vi "Configuration File.vi"(4 "Freq List File":path, 5 "Limit File":path, 6 "Configurtion File":path, 7 "Mode (F-Read)":bool, 8 "Error In":errorcluster, 9 "Limit":T1, 10 "Freq List In":cluster{"Freq":dbl, "Amp":dbl}[](array[cluster]), 11 "Configuration":T2={"PSU Setting"={"Channel Name"="1", "Source Delay (Sec)"=0.5, "Measurement:Sense"=1008, "voltage level"=0.0, "voltage level range"=20.0, "current limit"=0.02, "current limit range"=0.02, "resource name"="PSU"}, "Sweep Settings"={"Input Settings"={"IEPE min time to settle [s]"=0.0, "Responce Channel Settings"={"DSA response channel settings"={"coupling"=10045, "enable IEPE excitation"=FALSE, "IEPE current [mA]"=4.0}, "response channel info"={"sensor sensitivity"=1000.0, "engineering units"=1, "dB reference"=1.0, "custom label"="EU", "weighting filter"=0, "pregain"=0.0}, "AI response settings"={"response channel"="SOUNDACQ/ai1", "max value [V]"=10.0, "min value [V]"=-10.0, "terminal configuration"=-1}}, "Stimulus Channel Settings"={"AI stimulus settings"={"stimulus channel"="SOUNDACQ/ai0", "max value [V]"=2.0, "min value [V]"=-2.0, "terminal configuration"=-1}, "DSA stimulus channel settings"={"coupling"=10045, "enable IEPE excitation"=TRUE, "IEPE current [mA]"=4.0}, "stimulus channel info"={"sensor sensitivity"=11.4, "engineering units"=2, "dB reference"=2e-05, "custom label"="EU", "weighting filter"=0, "pregain"=0.0}}}, "Output Settings"={"AO source settings"={"excitation channel"="SOUNDACQ/ao0", "max value [V]"=10.0, "min value [V]"=-10.0, "terminal configuration"=-1}}}} {"Sweep Settings"."Output Settings"."AO source settings"."terminal configuration" items=["Default"=-1, "RSE"=10083, "Differential"=10106, "Pseudodifferential"=12529]; "Sweep Settings"."Output Settings"."AO source settings"."min value [V]" format="%0.2f"; "Sweep Settings"."Output Settings"."AO source settings"."max value [V]" format="%0.2f"; "Sweep Settings"."Input Settings"."Stimulus Channel Settings"."stimulus channel info"."pregain" format="%.2f"; "Sweep Settings"."Input Settings"."Stimulus Channel Settings"."stimulus channel info"."weighting filter" items=["Linear", "A-weighting", "B-weighting", "C-weighting", "ITU-R 468-4", "Dolby", "CCITT", "C-message", "Wb", "Wc", "Wd", "We", "Wf", "Wh", "Wj", "Wk", "Wm", "AES17 20 kHz lowpass", "AES17 40 kHz lowpass", "AES17 20 kHz highpass", "AES17 40 kHz highpass"]; "Sweep Settings"."Input Settings"."Stimulus Channel Settings"."stimulus channel info"."dB reference" format="%^.1e"; "Sweep Settings"."Input Settings"."Stimulus Channel Settings"."stimulus channel info"."engineering units" items=["custom..."=0, "V"=1, "A"=21, "C"=30, "pC"=31, "s"=32, "-"=29, "Pa"=2, "N"=20, "g"=3, "m/s^2"=4, "m/s"=5, "m"=6, "mm/s"=12, "mm"=13, "micron/s"=14, "micron"=15, "in/s^2"=7, "in/s"=8, "in"=9, "mil/s"=10, "mil"=11, "rad/s^2"=16, "rad/s"=17, "rad"=18, "deg/s^2"=26, "deg/s"=27, "deg"=28, "RPM"=22, "cycle/s^2"=23, "Hz"=24, "cycle"=25, "strain"=19]; "Sweep Settings"."Input Settings"."Stimulus Channel Settings"."stimulus channel info"."sensor sensitivity" format="%#_5f"; "Sweep Settings"."Input Settings"."Stimulus Channel Settings"."DSA stimulus channel settings"."IEPE current [mA]" format="%.1f"; "Sweep Settings"."Input Settings"."Stimulus Channel Settings"."DSA stimulus channel settings"."coupling" items=["AC"=10045, "DC"=10050, "GND"=10066]; "Sweep Settings"."Input Settings"."Stimulus Channel Settings"."AI stimulus settings"."terminal configuration" items=["Default"=-1, "RSE"=10083, "NRSE"=10078, "Differential"=10106, "Pseudodifferential"=12529]; "Sweep Settings"."Input Settings"."Stimulus Channel Settings"."AI stimulus settings"."min value [V]" format="%.2f"; "Sweep Settings"."Input Settings"."Stimulus Channel Settings"."AI stimulus settings"."max value [V]" format="%.2f"; "Sweep Settings"."Input Settings"."Responce Channel Settings"."AI response settings"."terminal configuration" items=["Default"=-1, "RSE"=10083, "NRSE"=10078, "Differential"=10106, "Pseudodifferential"=12529]; "Sweep Settings"."Input Settings"."Responce Channel Settings"."AI response settings"."min value [V]" format="%.2f"; "Sweep Settings"."Input Settings"."Responce Channel Settings"."AI response settings"."max value [V]" format="%.2f"; "Sweep Settings"."Input Settings"."Responce Channel Settings"."response channel info"."pregain" format="%.2f"; "Sweep Settings"."Input Settings"."Responce Channel Settings"."response channel info"."weighting filter" items=["Linear", "A-weighting", "B-weighting", "C-weighting", "ITU-R 468-4", "Dolby", "CCITT", "C-message", "Wb", "Wc", "Wd", "We", "Wf", "Wh", "Wj", "Wk", "Wm", "AES17 20 kHz lowpass", "AES17 40 kHz lowpass", "AES17 20 kHz highpass", "AES17 40 kHz highpass"]; "Sweep Settings"."Input Settings"."Responce Channel Settings"."response channel info"."dB reference" format="%^.1e"; "Sweep Settings"."Input Settings"."Responce Channel Settings"."response channel info"."engineering units" items=["custom..."=0, "V"=1, "A"=21, "C"=30, "pC"=31, "s"=32, "-"=29, "Pa"=2, "N"=20, "g"=3, "m/s^2"=4, "m/s"=5, "m"=6, "mm/s"=12, "mm"=13, "micron/s"=14, "micron"=15, "in/s^2"=7, "in/s"=8, "in"=9, "mil/s"=10, "mil"=11, "rad/s^2"=16, "rad/s"=17, "rad"=18, "deg/s^2"=26, "deg/s"=27, "deg"=28, "RPM"=22, "cycle/s^2"=23, "Hz"=24, "cycle"=25, "strain"=19]; "Sweep Settings"."Input Settings"."Responce Channel Settings"."response channel info"."sensor sensitivity" format="%#_5f"; "Sweep Settings"."Input Settings"."Responce Channel Settings"."DSA response channel settings"."IEPE current [mA]" format="%.1f"; "Sweep Settings"."Input Settings"."Responce Channel Settings"."DSA response channel settings"."coupling" items=["AC"=10045, "DC"=10050, "GND"=10066]; "Sweep Settings"."Input Settings"."IEPE min time to settle [s]" format="%.1f"; "PSU Setting"."current limit range" format="%_6p"; "PSU Setting"."current limit" format="%_6p"; "PSU Setting"."voltage level range" format="%_6p"; "PSU Setting"."voltage level" format="%_6p"; "PSU Setting"."Measurement:Sense" items=["Local"=1008, "Remote"=1009]; "PSU Setting"."Source Delay (Sec)" format="%_6p"}) -> (0 "Error Out":errorcluster, 1 "Limit Out":T1, 2 "Freq List Out":cluster{"Freq":dbl, "Amp":dbl}[](array[cluster]), 3 "value":T2={"PSU Setting"={"Channel Name"="1", "Source Delay (Sec)"=0.5, "Measurement:Sense"=1008, "voltage level"=0.0, "voltage level range"=20.0, "current limit"=0.02, "current limit range"=0.02, "resource name"="PSU"}, "Sweep Settings"={"Input Settings"={"IEPE min time to settle [s]"=0.0, "Responce Channel Settings"={"DSA response channel settings"={"coupling"=10045, "enable IEPE excitation"=FALSE, "IEPE current [mA]"=4.0}, "response channel info"={"sensor sensitivity"=1000.0, "engineering units"=1, "dB reference"=1.0, "custom label"="EU", "weighting filter"=0, "pregain"=0.0}, "AI response settings"={"response channel"="SOUNDACQ/ai1", "max value [V]"=10.0, "min value [V]"=-10.0, "terminal configuration"=-1}}, "Stimulus Channel Settings"={"AI stimulus settings"={"stimulus channel"="SOUNDACQ/ai0", "max value [V]"=2.0, "min value [V]"=-2.0, "terminal configuration"=-1}, "DSA stimulus channel settings"={"coupling"=10045, "enable IEPE excitation"=TRUE, "IEPE current [mA]"=4.0}, "stimulus channel info"={"sensor sensitivity"=11.4, "engineering units"=2, "dB reference"=2e-05, "custom label"="EU", "weighting filter"=0, "pregain"=0.0}}}, "Output Settings"={"AO source settings"={"excitation channel"="SOUNDACQ/ao0", "max value [V]"=10.0, "min value [V]"=-10.0, "terminal configuration"=-1}}}} {"Sweep Settings"."Output Settings"."AO source settings"."terminal configuration" items=["Default"=-1, "RSE"=10083, "Differential"=10106, "Pseudodifferential"=12529]; "Sweep Settings"."Output Settings"."AO source settings"."min value [V]" format="%0.2f"; "Sweep Settings"."Output Settings"."AO source settings"."max value [V]" format="%0.2f"; "Sweep Settings"."Input Settings"."Stimulus Channel Settings"."stimulus channel info"."pregain" format="%.2f"; "Sweep Settings"."Input Settings"."Stimulus Channel Settings"."stimulus channel info"."weighting filter" items=["Linear", "A-weighting", "B-weighting", "C-weighting", "ITU-R 468-4", "Dolby", "CCITT", "C-message", "Wb", "Wc", "Wd", "We", "Wf", "Wh", "Wj", "Wk", "Wm", "AES17 20 kHz lowpass", "AES17 40 kHz lowpass", "AES17 20 kHz highpass", "AES17 40 kHz highpass"]; "Sweep Settings"."Input Settings"."Stimulus Channel Settings"."stimulus channel info"."dB reference" format="%^.1e"; "Sweep Settings"."Input Settings"."Stimulus Channel Settings"."stimulus channel info"."engineering units" items=["custom..."=0, "V"=1, "A"=21, "C"=30, "pC"=31, "s"=32, "-"=29, "Pa"=2, "N"=20, "g"=3, "m/s^2"=4, "m/s"=5, "m"=6, "mm/s"=12, "mm"=13, "micron/s"=14, "micron"=15, "in/s^2"=7, "in/s"=8, "in"=9, "mil/s"=10, "mil"=11, "rad/s^2"=16, "rad/s"=17, "rad"=18, "deg/s^2"=26, "deg/s"=27, "deg"=28, "RPM"=22, "cycle/s^2"=23, "Hz"=24, "cycle"=25, "strain"=19]; "Sweep Settings"."Input Settings"."Stimulus Channel Settings"."stimulus channel info"."sensor sensitivity" format="%#_5f"; "Sweep Settings"."Input Settings"."Stimulus Channel Settings"."DSA stimulus channel settings"."IEPE current [mA]" format="%.1f"; "Sweep Settings"."Input Settings"."Stimulus Channel Settings"."DSA stimulus channel settings"."coupling" items=["AC"=10045, "DC"=10050, "GND"=10066]; "Sweep Settings"."Input Settings"."Stimulus Channel Settings"."AI stimulus settings"."terminal configuration" items=["Default"=-1, "RSE"=10083, "NRSE"=10078, "Differential"=10106, "Pseudodifferential"=12529]; "Sweep Settings"."Input Settings"."Stimulus Channel Settings"."AI stimulus settings"."min value [V]" format="%.2f"; "Sweep Settings"."Input Settings"."Stimulus Channel Settings"."AI stimulus settings"."max value [V]" format="%.2f"; "Sweep Settings"."Input Settings"."Responce Channel Settings"."AI response settings"."terminal configuration" items=["Default"=-1, "RSE"=10083, "NRSE"=10078, "Differential"=10106, "Pseudodifferential"=12529]; "Sweep Settings"."Input Settings"."Responce Channel Settings"."AI response settings"."min value [V]" format="%.2f"; "Sweep Settings"."Input Settings"."Responce Channel Settings"."AI response settings"."max value [V]" format="%.2f"; "Sweep Settings"."Input Settings"."Responce Channel Settings"."response channel info"."pregain" format="%.2f"; "Sweep Settings"."Input Settings"."Responce Channel Settings"."response channel info"."weighting filter" items=["Linear", "A-weighting", "B-weighting", "C-weighting", "ITU-R 468-4", "Dolby", "CCITT", "C-message", "Wb", "Wc", "Wd", "We", "Wf", "Wh", "Wj", "Wk", "Wm", "AES17 20 kHz lowpass", "AES17 40 kHz lowpass", "AES17 20 kHz highpass", "AES17 40 kHz highpass"]; "Sweep Settings"."Input Settings"."Responce Channel Settings"."response channel info"."dB reference" format="%^.1e"; "Sweep Settings"."Input Settings"."Responce Channel Settings"."response channel info"."engineering units" items=["custom..."=0, "V"=1, "A"=21, "C"=30, "pC"=31, "s"=32, "-"=29, "Pa"=2, "N"=20, "g"=3, "m/s^2"=4, "m/s"=5, "m"=6, "mm/s"=12, "mm"=13, "micron/s"=14, "micron"=15, "in/s^2"=7, "in/s"=8, "in"=9, "mil/s"=10, "mil"=11, "rad/s^2"=16, "rad/s"=17, "rad"=18, "deg/s^2"=26, "deg/s"=27, "deg"=28, "RPM"=22, "cycle/s^2"=23, "Hz"=24, "cycle"=25, "strain"=19]; "Sweep Settings"."Input Settings"."Responce Channel Settings"."response channel info"."sensor sensitivity" format="%#_5f"; "Sweep Settings"."Input Settings"."Responce Channel Settings"."DSA response channel settings"."IEPE current [mA]" format="%.1f"; "Sweep Settings"."Input Settings"."Responce Channel Settings"."DSA response channel settings"."coupling" items=["AC"=10045, "DC"=10050, "GND"=10066]; "Sweep Settings"."Input Settings"."IEPE min time to settle [s]" format="%.1f"; "PSU Setting"."current limit range" format="%_6p"; "PSU Setting"."current limit" format="%_6p"; "PSU Setting"."voltage level range" format="%_6p"; "PSU Setting"."voltage level" format="%_6p"; "PSU Setting"."Measurement:Sense" items=["Local"=1008, "Remote"=1009]; "PSU Setting"."Source Delay (Sec)" format="%_6p"})   [LabVIEW 2018]
uses:
  Types/ConfigurationType.ctl
  PowerSupply4110/Type/SupplyConfig.ctl
  Microfontest/Peiker_Stepped Sweep Settings.ctl
  <vilib>/addons/_NISVFA/_Shared subVIs/Controls/svc_DSA Channel Settings.ctl
  <vilib>/addons/_NISVFA/_Shared subVIs/Controls/svc_Channel Info.ctl
  <vilib>/addons/_NISVFA/_Shared subVIs/Controls/svc_Engineering Units Text Ring.ctl
  <vilib>/addons/_NISVFA/_Shared subVIs/Controls/svc_Weighting Filter Text Ring.ctl
  Types/LimitType.ctl
  <vilib>/Utility/xml.llb/Read From XML File(string).vi
  <vilib>/Utility/file.llb/Read Delimited Spreadsheet (DBL).vi
  <vilib>/Utility/xml.llb/Write to XML File(string).vi
  <vilib>/Utility/file.llb/Write Delimited Spreadsheet (DBL).vi
panel:
  # "Einstellungen"
  # "Einstellungen"
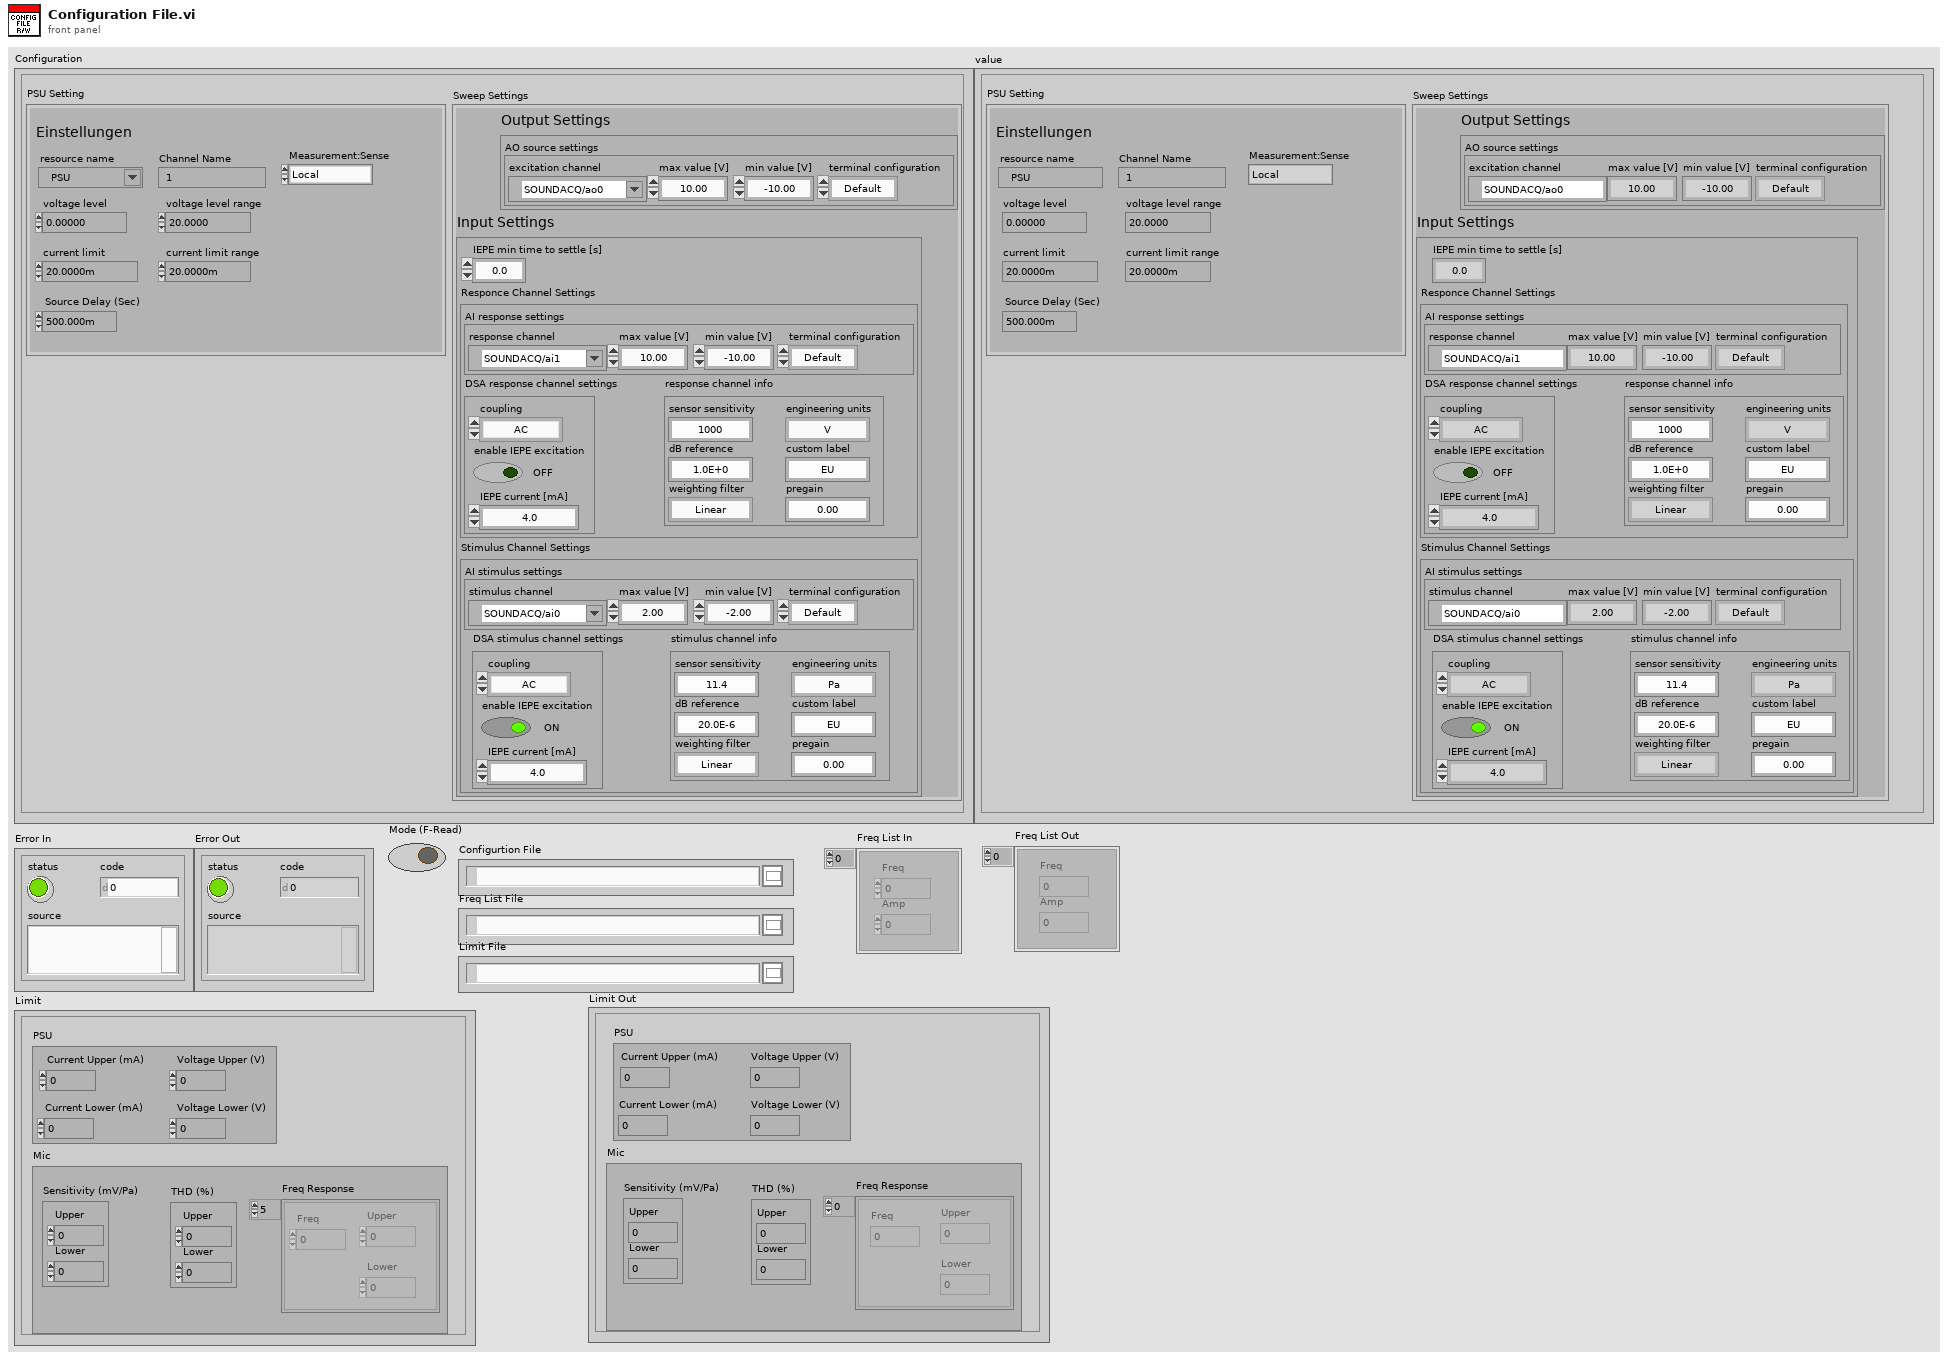
[diagram p1: front panel]
types:
  T1 = typedef "LimitType.ctl" = cluster{"PSU":cluster{"Current Lower (mA)":dbl, "Current Upper (mA)":dbl, "Voltage Lower (V)":dbl, "Voltage Upper (V)":dbl}, "Mic":cluster{"Sensitivity (mV/Pa)":cluster{"Lower":dbl, "Upper":dbl}, "THD (%)":cluster{"Lower":dbl, "Upper":dbl}, "Freq Response":cluster{"Freq":dbl, "Upper":dbl, "Lower":dbl}[]}}
  T2 = typedef "ConfigurationType.ctl" = cluster{"PSU Setting":T3, "Sweep Settings":T4}
  T3 = typedef "SupplyConfig.ctl" = cluster{"Channel Name":string, "Source Delay (Sec)":dbl, "Measurement:Sense":i32, "voltage level":dbl, "voltage level range":dbl, "current limit":dbl, "current limit range":dbl, "resource name":refnum<k15>}
  T4 = typedef "Peiker_Stepped Sweep Settings.ctl" = cluster{"Input Settings":cluster{"IEPE min time to settle [s]":dbl, "Responce Channel Settings":cluster{"DSA response channel settings":T5, "response channel info":T6, "AI response settings":cluster{"response channel":tag, "max value [V]":dbl, "min value [V]":dbl, "terminal configuration":i32}}, "Stimulus Channel Settings":cluster{"AI stimulus settings":cluster{"stimulus channel":tag, "max value [V]":dbl, "min value [V]":dbl, "terminal configuration":i32}, "DSA stimulus channel settings":T5, "stimulus channel info":T6}}, "Output Settings":cluster{"AO source settings":cluster{"excitation channel":tag, "max value [V]":dbl, "min value [V]":dbl, "terminal configuration":i32}}}
  T5 = typedef "svc_DSA Channel Settings.ctl" = cluster{"coupling":i32, "enable IEPE excitation":bool, "IEPE current [mA]":dbl}
  T6 = typedef "svc_Channel Info.ctl" = cluster{"sensor sensitivity":dbl, "engineering units":T7, "dB reference":dbl, "custom label":string, "weighting filter":T8, "pregain":dbl}
  T7 = typedef "svc_Engineering Units Text Ring.ctl" = u16
  T8 = typedef "svc_Weighting Filter Text Ring.ctl" = u16
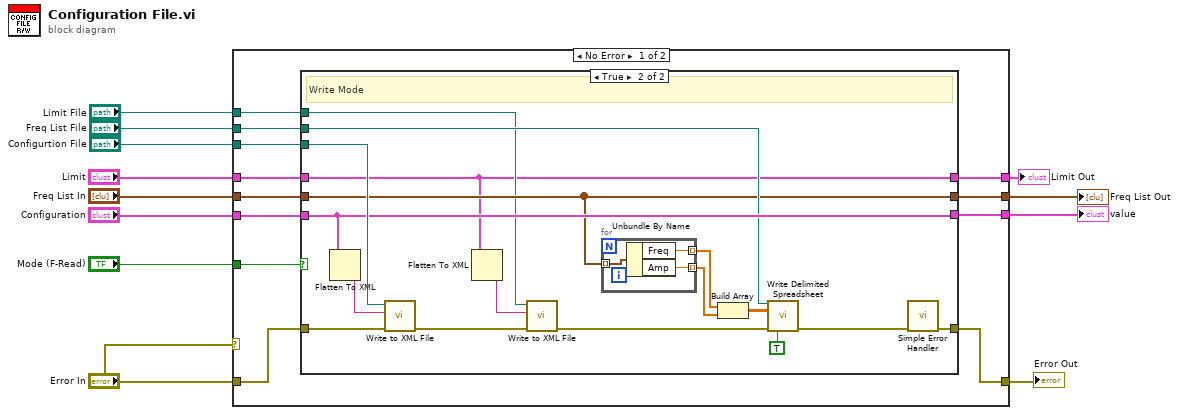
[diagram p0: block diagram]
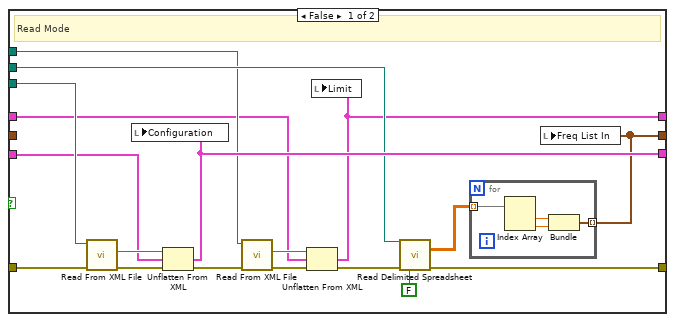
[diagram p2: hidden frame]
diagram:
  n1 = case shown="No Error" "Error In" {
    tunnel: "Error In" -> [w21 w70]
    tunnel: "Configuration" -> [w24 w69]
    tunnel: "Mode (F-Read)" -> [w23 _]
    tunnel: "Configurtion File" -> [w22 _]
    tunnel: [w20 w70] -> w8
    tunnel: [w19 w69] -> w7
    tunnel: "Freq List File" -> [w18 _]
    tunnel: "Freq List In" -> [w17 w68]
    tunnel: [w16 w68] -> w4
    tunnel: "Limit" -> [w15 w67]
    tunnel: "Limit File" -> [w14 _]
    tunnel: [w13 w67] -> w1
    frame No Error {
      n2 = case shown="True" w23 {
        tunnel: w24 -> [w38 w59]
        tunnel: w22 -> [w42 w62]
        tunnel: w21 -> [w41 w63]
        tunnel: [w35 w60] -> w20
        tunnel: [w37 w59] -> w19
        tunnel: w18 -> [w34 w53]
        tunnel: w17 -> [_ w52]
        tunnel: [w32 w52] -> w16
        tunnel: w15 -> [w27 w47]
        tunnel: w14 -> [w28 w48]
        tunnel: [w25 w47] -> w13
        frame False {
          # "Read Mode"
          n3 = call-poly <vilib>:"Read From XML File.vi"("error in (no error)"=w41, "XML File Path"=w42) -> ("error out"=w39:errorcluster, "XML Elements"=w40:string)  [unwired: 7 in, 1 out]
          n4 = Unflatten From XML(xml string=w40, type=w38, error in (no error)=w39) -> (value=w37:T2, error out=w29:errorcluster)
          n5 = local write "Configuration"(w37) -> ()
          n6 = call-poly <vilib>:"Read From XML File.vi"("error in (no error)"=w29, "XML File Path"=w28) -> ("error out"=w31:errorcluster, "XML Elements"=w30:string)  [unwired: 7 in, 1 out]
          n7 = Unflatten From XML(xml string=w30, type=w27, error in (no error)=w31) -> (value=w25:T1, error out=w26:errorcluster)
          n8 = local write "Limit"(w25) -> ()
          n9 = call-poly <vilib>:"Read Delimited Spreadsheet.vi"("file path (dialog if empty)"=w34, "error in (no error)"=w26, "transpose? (F)"=FALSE) -> ("all rows"=w33:dbl[][], "error out"=w35:errorcluster)  [unwired: 7 in, 4 out]
          n10 = for {
            tunnel: w33 -> [w46] mode=indexing
            tunnel: [w43] -> w32 mode=indexing
            n11 = Index Array(array=w46) -> (element #1=w45:dbl, element #2=w44:dbl)  [unwired: 2 in]
            n12 = Bundle("Numeric"=w45, "Numeric"=w44) -> (w43:cluster{"Numeric":dbl, "Numeric":dbl})  [unwired: 1 in]
          }
          n13 = local write "Freq List In"(w32) -> ()
        }
        frame True {
          # "Write Mode"
          n14 = Flatten To XML(anything=w59) -> (xml string=w61:string)
          n15 = call-poly <vilib>:"Write to XML File.vi"("error in (no error)"=w63, "XML Input"=w61, "XML File Path"=w62) -> ("error out"=w50:errorcluster)  [unwired: 6 in, 2 out]
          n16 = Flatten To XML(anything=w47) -> (xml string=w51:string)
          n17 = call-poly <vilib>:"Write to XML File.vi"("error in (no error)"=w50, "XML Input"=w51, "XML File Path"=w48) -> ("error out"=w49:errorcluster)  [unwired: 6 in, 2 out]
          n18 = for {
            tunnel: w52 -> [w66] mode=indexing
            tunnel: [w65] -> w56 mode=indexing
            tunnel: [w64] -> w57 mode=indexing
            n19 = Unbundle By Name(w66) -> ("Freq"=w65:dbl, "Amp"=w64:dbl)
          }
          n20 = Build Array(w56, w57) -> (w58:dbl[][])
          n21 = call-poly <vilib>:"Write Delimited Spreadsheet.vi"("file path (dialog if empty)"=w53, "2D data"=w58, "error in (no error)"=w49, "transpose? (no:F)"=TRUE) -> ("error out"=w54:errorcluster)  [unwired: 10 in, 1 out]
          n22 = call <vilib>:"Simple Error Handler.vi"("error in (no error)"=w54) -> ("error out"=w60:errorcluster)  [unwired: 4 in, 4 out]
        }
      }
    }
    frame Error {
    }
  }
  "Error Out" <- w8
  "value" <- w7
  "Freq List Out" <- w4
  "Limit Out" <- w1
